vi "TrendsD05.vi"() -> ()   [LabVIEW 2019, in "D05.lvlib"]
uses:
  D05.lvlib
  <vilib>/measure/mamon.llb/Trigger Detection for 1 Channel.vi
  <vilib>/measure/NI_MAPro.lvlib
panel:
  out "No Change":bool
  out "Sudden Change":bool
  out "Decrease":bool
  out "Increase":bool
  out "Previous  ES":dbl
  out "Present  Speed":dbl
  out "Present Error":dbl format="%#.2g"
  out "Previous Error":dbl
  out "Previous  Speed":dbl
  out "Previous PW":dbl caption="Control Information"
  out "Pulse Trends":waveform(i16)[](graph) caption="Waveform Chart - Dark"
  in  "Close":bool
  out "disc name":string="Disc 05 Trends"
  out "dsgs":string="DSGS"
  out "Speed Trend":waveform(dbl)(graph) caption="Waveform Chart - Dark"
  out "Average Trend":waveform(dbl)[](graph) caption="Waveform Chart - Dark"
  out "Live Trend":waveform(dbl)[](graph) caption="Waveform Chart - Dark"
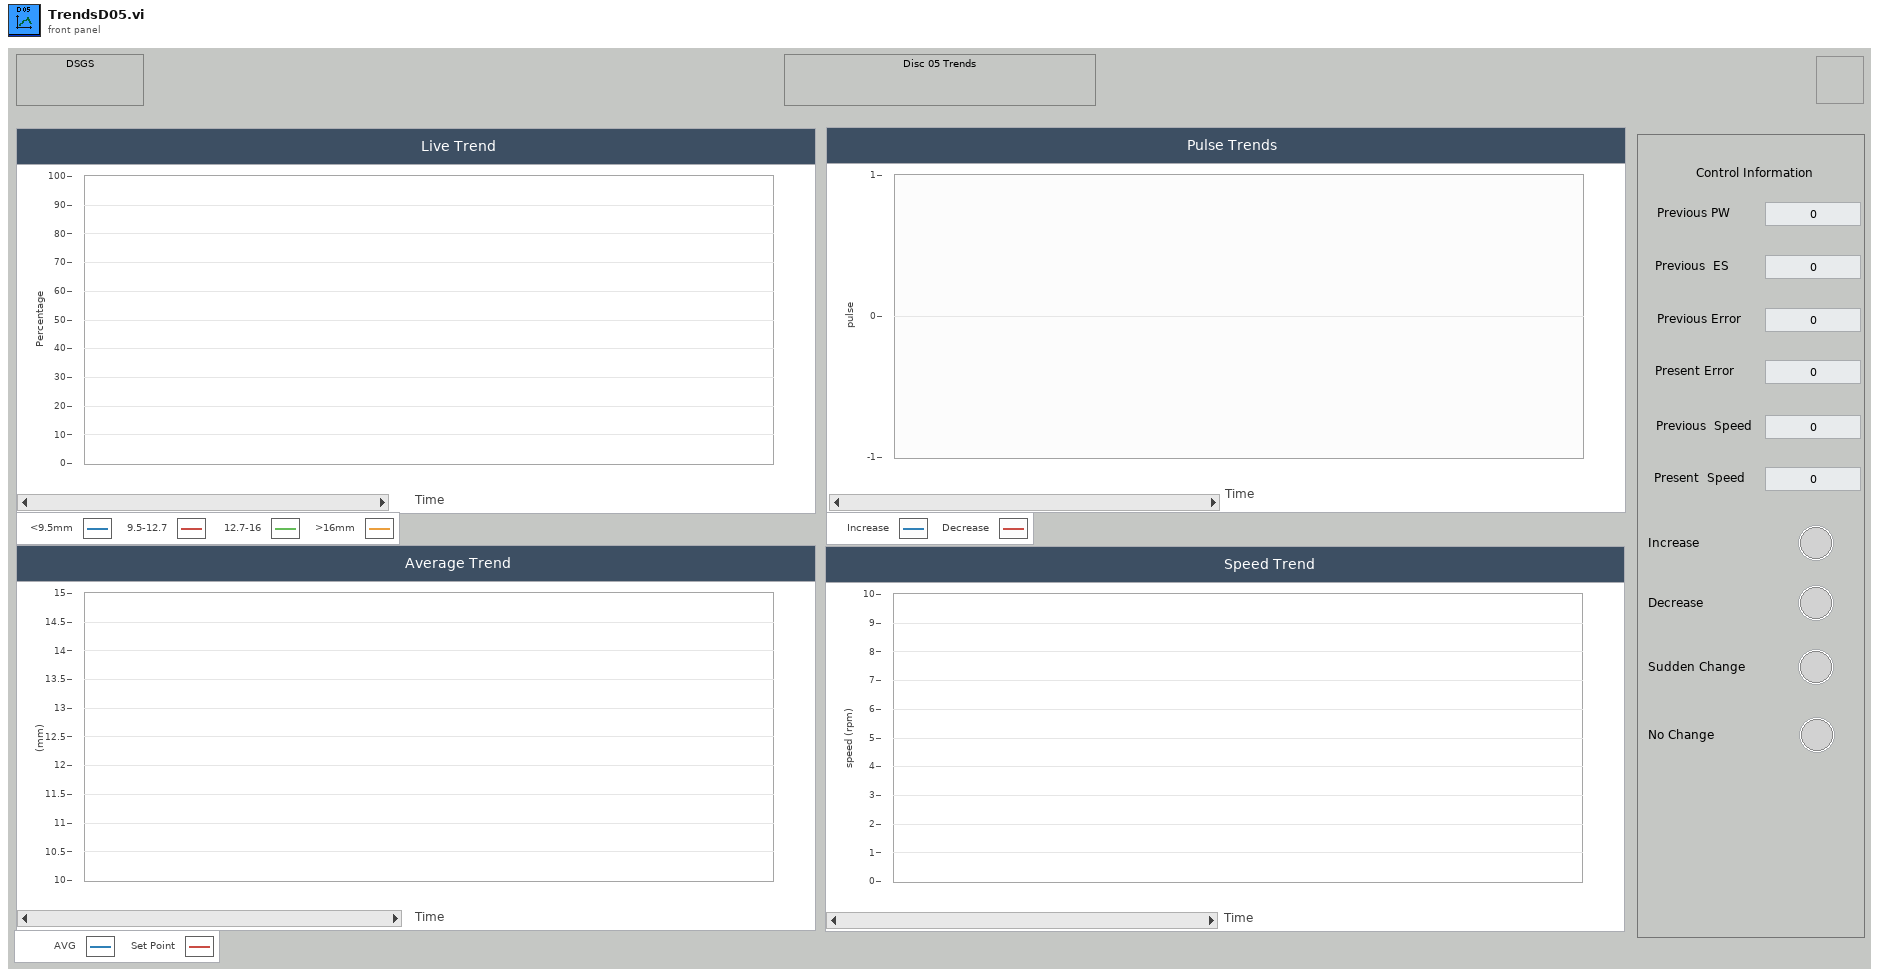
[diagram p1: front panel]
types:
  T1 = cluster{"decrease D30":bool, "increase D30":bool, "no change D30":bool, "sudden change D30":bool, "last error 30":dbl, "previouse speed D30":dbl, "pulse width D30":dbl, "slope D30":dbl}
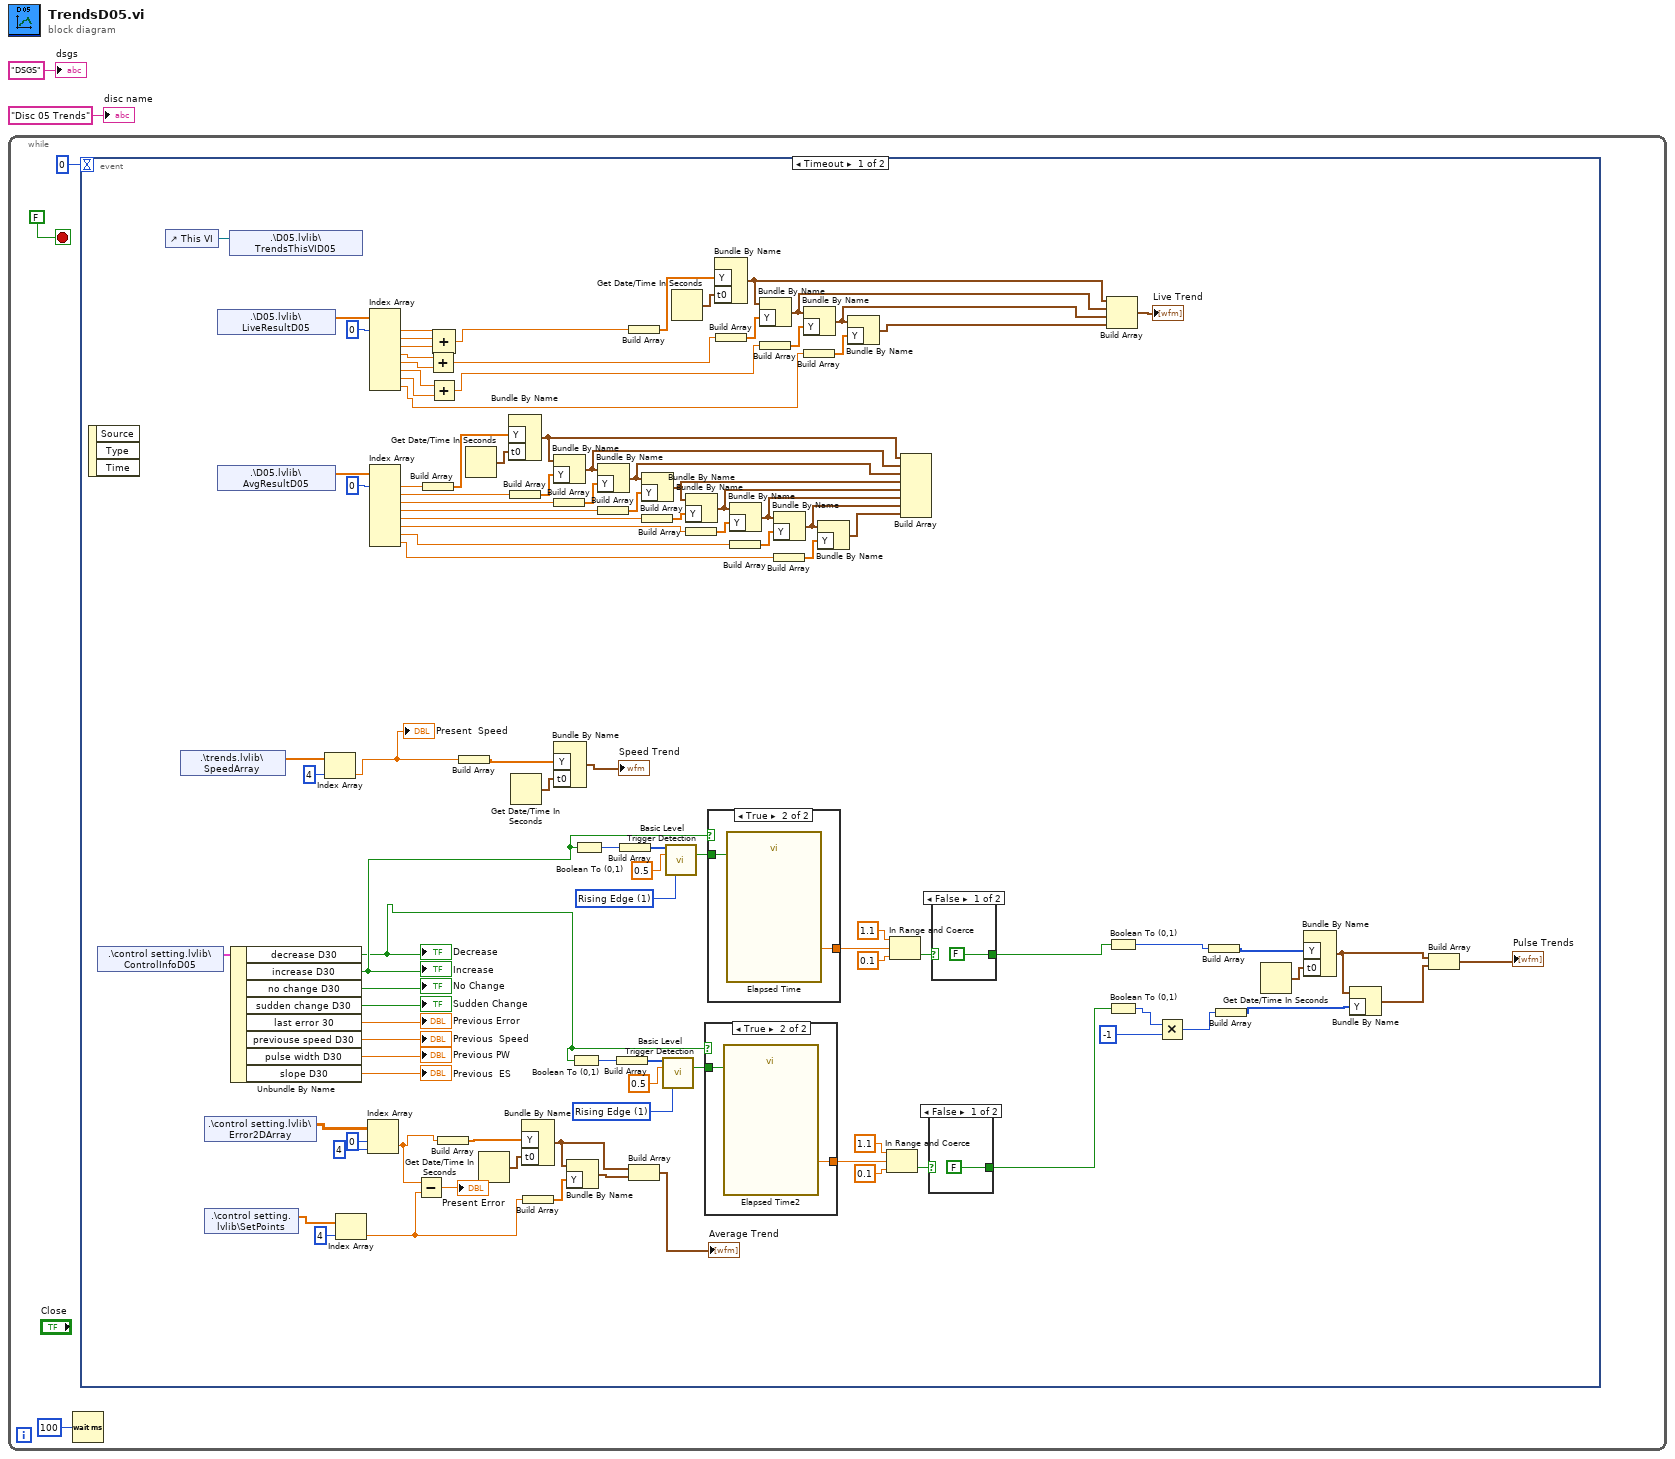
[diagram p0: block diagram]
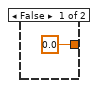
[diagram p2: hidden frame]
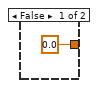
[diagram p4: hidden frame]
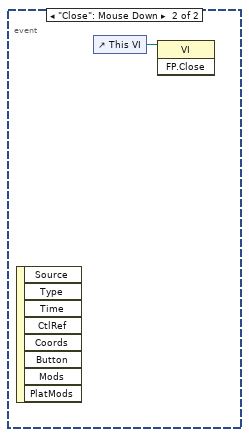
[diagram p6: hidden frame]
diagram:
  n1 = while {
    stop <- FALSE stop-if-true
    n2 = Wait (ms)(milliseconds to wait=u32 100) -> ()  [unwired: 1 out]
    n3 = event shown="[0] Timeout" {
      selector: _ -> [_ _]
      dyn-events: _ -> [_ _]
      timeout: 0 -> [_ _]
      event Timeout {
        w34 = u16 1 items=["Falling Edge", "Rising Edge"] ("trigger slope")
        w39 = u16 1 items=["Falling Edge", "Rising Edge"] ("trigger slope")
        n4 = event-data() -> ()  [unwired: 1 in, 3 out]
        n5 = shared-variable ".\\control setting.lvlib\\ControlInfoD05"() -> (w60:T1)  [unwired: 1 in, 1 out]
        n6 = control-ref of="This VI"() -> (w76:refnum<vi>)
        n7 = shared-variable ".\\trends.lvlib\\SpeedArray"() -> (w65:dbl[])  [unwired: 1 in, 1 out]
        n8 = shared-variable ".\\control setting.lvlib\\Error2DArray"() -> (w53:dbl[][])  [unwired: 1 in, 1 out]
        n9 = shared-variable ".\\control setting.lvlib\\SetPoints"() -> (w50:dbl[])  [unwired: 1 in, 1 out]
        n10 = shared-variable ".\\D05.lvlib\\LiveResultD05"() -> (w115:dbl[])  [unwired: 1 in, 1 out]
        n11 = shared-variable ".\\D05.lvlib\\AvgResultD05"() -> (w82:dbl[])  [unwired: 1 in, 1 out]
        n12 = shared-variable ".\\D05.lvlib\\TrendsThisVID05"(w76) -> ()  [unwired: 1 in, 1 out]
        n13 = Unbundle By Name(w60) -> ("decrease D30"=w26:bool, "increase D30"=w37:bool, "no change D30"=→"No Change":bool, "sudden change D30"=→"Sudden Change":bool, "last error 30"=→"Previous Error":dbl, "previouse speed D30"=→"Previous  Speed":dbl, "pulse width D30"=→"Previous PW":dbl, "slope D30"=→"Previous  ES":dbl)
        "Increase" <- w37
        "Decrease" <- w26
        n14 = Index Array(array=w65, index=4) -> (element=w47:dbl)
        "Present  Speed" <- w47
        n15 = Index Array(array=w50, index=4) -> (element=w9:dbl)
        n16 = Index Array(array=w53, index (row)=0, index (col)=4 ("disabled index (col)")) -> (element=w10:dbl)
        n17 = Index Array(array=w115, index #1=0 ("index")) -> (element #1=w24:dbl, element #2=w23:dbl, element #3=w22:dbl, element #4=w20:dbl, element #5=w19:dbl, element #6=w18:dbl, element #7=w17:dbl, element #8=w14:dbl)  [unwired: 7 in]
        n18 = Index Array(array=w82, index #1=0 ("index")) -> (element #1=w92:dbl, element #2=w93:dbl, element #3=w95:dbl, element #4=w97:dbl, element #5=w98:dbl, element #6=w100:dbl, element #7=w102:dbl, element #8=w79:dbl)  [unwired: 7 in]
        n19 = Subtract(x=w10, y=w9) -> (x-y=→"Present Error":dbl)
        n20 = Build Array(w92) -> (w103:dbl[])
        n21 = Add(x=w20, y=w19) -> (x+y=w16:dbl)
        n22 = Add(x=w18, y=w17) -> (x+y=w15:dbl)
        n23 = Compound Arithmetic op=ADD(w24, w23, w22) -> (w21:dbl)
        n24 = Build Array(w10) -> (w13:dbl[])
        n25 = Build Array(w47) -> (w63:dbl[])
        n26 = Get Date/Time In Seconds() -> (seconds since 1Jan1904=w85:timestamp)
        n27 = Get Date/Time In Seconds() -> (seconds since 1Jan1904=w11:timestamp)
        n28 = Bundle By Name("Y"=w103, "t0"=w85) -> (w91:waveform(dbl))  [unwired: 1 in]
        n29 = Build Array(w93) -> (w94:dbl[])
        n30 = Get Date/Time In Seconds() -> (seconds since 1Jan1904=w62:timestamp)
        n31 = Bundle By Name("Y"=w13, "t0"=w11) -> (w8:waveform(dbl))  [unwired: 1 in]
        n32 = Build Array(w9) -> (w12:dbl[])
        n33 = Bundle By Name(cluster=w91, "Y"=w94) -> (w90:waveform(dbl))
        n34 = Build Array(w95) -> (w96:dbl[])
        n35 = Bundle By Name("Y"=w63, "t0"=w62) -> (→"Speed Trend":waveform(dbl))  [unwired: 1 in]
        n36 = Bundle By Name(cluster=w8, "Y"=w12) -> (w7:waveform(dbl))
        n37 = Boolean To (0,1)(Boolean=w26) -> (0, 1=w31:i16)
        n38 = Boolean To (0,1)(Boolean=w37) -> (0, 1=w42:i16)
        n39 = Bundle By Name(cluster=w90, "Y"=w96) -> (w89:waveform(dbl))
        n40 = Build Array(w97) -> (w84:dbl[])
        n41 = Build Array(w31) -> (w32:i16[])
        n42 = Build Array(w42) -> (w41:i16[])
        n43 = Build Array(w21) -> (w105:dbl[])
        n44 = Build Array(w8, w7) -> (→"Average Trend":waveform(dbl)[])
        n45 = Bundle By Name(cluster=w89, "Y"=w84) -> (w88:waveform(dbl))
        n46 = Build Array(w98) -> (w99:dbl[])
        n47 = call-poly <vilib>:"Basic Level Trigger Detection.vi"("signal in"=w32, "level"=0.5, "trigger slope"=w34) -> ("trigger detected?"=w35:bool)  [unwired: 10 in, 2 out]
        n48 = call-poly <vilib>:"Basic Level Trigger Detection.vi"("signal in"=w41, "level"=0.5, "trigger slope"=w39) -> ("trigger detected?"=w38:bool)  [unwired: 10 in, 2 out]
        n49 = Get Date/Time In Seconds() -> (seconds since 1Jan1904=w112:timestamp)
        n50 = Bundle By Name(cluster=w88, "Y"=w99) -> (w87:waveform(dbl))
        n51 = Build Array(w100) -> (w101:dbl[])
        n52 = case shown="True" w26 {
          tunnel: [0.0 ("Elapsed Time (s)") w117] -> w27
          tunnel: w35 -> [_ w118]
          frame False {
          }
          frame True {
            n53 = call "Elapsed Time2"("Reset"=w118) -> ("Elapsed Time (s)"=w117:dbl)  [unwired: 11 in, 7 out]
          }
        }
        n54 = case shown="True" w37 {
          tunnel: [0.0 ("Elapsed Time (s)") w122] -> w46
          tunnel: w38 -> [_ w123]
          frame False {
          }
          frame True {
            n55 = call "Elapsed Time"("Reset"=w123) -> ("Elapsed Time (s)"=w122:dbl)  [unwired: 11 in, 7 out]
          }
        }
        n56 = Bundle By Name("Y"=w105, "t0"=w112) -> (w108:waveform(dbl))  [unwired: 1 in]
        n57 = Build Array(w16) -> (w107:dbl[])
        n58 = Bundle By Name(cluster=w87, "Y"=w101) -> (w86:waveform(dbl))
        n59 = Build Array(w102) -> (w104:dbl[])
        n60 = Bundle By Name(cluster=w108, "Y"=w107) -> (w109:waveform(dbl))
        n61 = Build Array(w15) -> (w106:dbl[])
        n62 = Bundle By Name(cluster=w86, "Y"=w104) -> (w80:waveform(dbl))
        n63 = Build Array(w79) -> (w81:dbl[])
        n64 = Bundle By Name(cluster=w109, "Y"=w106) -> (w110:waveform(dbl))
        n65 = Build Array(w14) -> (w113:dbl[])
        n66 = Bundle By Name(cluster=w80, "Y"=w81) -> (w78:waveform(dbl))
        n67 = Bundle By Name(cluster=w110, "Y"=w113) -> (w111:waveform(dbl))
        n68 = In Range and Coerce(upper limit=1.1, x=w27, lower limit=0.1) -> (In Range?=w30:bool)  [unwired: 1 out]
        n69 = In Range and Coerce(upper limit=1.1, x=w46, lower limit=0.1) -> (In Range?=w43:bool)  [unwired: 1 out]
        n70 = Build Array(w91, w90, w89, w88, w87, w86, w80, w78) -> ()  [unwired: 1 out]
        n71 = case shown="False" w30 {
          selector: w30 -> [_ w120]
          tunnel: [FALSE w120] -> w25
          frame False {
          }
          frame True {
          }
        }
        n72 = case shown="False" w43 {
          selector: w43 -> [_ w125]
          tunnel: [FALSE w125] -> w36
          frame False {
          }
          frame True {
          }
        }
        n73 = Build Array(w108, w109, w110, w111) -> (→"Live Trend":waveform(dbl)[])
        n74 = Boolean To (0,1)(Boolean=w36) -> (0, 1=w73:i16)
        n75 = Boolean To (0,1)(Boolean=w25) -> (0, 1=w69:i16)
        n76 = Multiply(x=w69, y=i16 -1 ("0, 1")) -> (x*y=w67:i16)
        n77 = Build Array(w73) -> (w74:i16[])
        n78 = Build Array(w67) -> (w72:i16[])
        n79 = Get Date/Time In Seconds() -> (seconds since 1Jan1904=w75:timestamp)
        n80 = Bundle By Name("Y"=w74, "t0"=w75) -> (w71:waveform(i16))  [unwired: 1 in]
        n81 = Bundle By Name(cluster=w71, "Y"=w72) -> (w70:waveform(i16))
        n82 = Build Array(w71, w70) -> (→"Pulse Trends":waveform(i16)[])
      }
      event "Close": Mouse Down {
        n83 = event-data() -> ()  [unwired: 1 in, 8 out]
        n84 = control-ref of="This VI"() -> (w126:refnum<vi>)
        n85 = invoke class="VI" method="FP.Close"(reference=w126) -> ()  [unwired: 2 in, 3 out]
      }
    }
  }
  "dsgs" <- "DSGS" ("dsgs")
  "disc name" <- "Disc 05 Trends" ("disc name")
